vi "Write SA Pin.vi"(8 "error in (no error)":errorcluster, 10 "SA Pin":string, 11 "SpecAn_IM3 in":refnum<class "SpecAn_IM3.lvclass">) -> (0 "error out":errorcluster, 3 "SpecAn_IM3 out":refnum<class "SpecAn_IM3.lvclass">)   [LabVIEW 2018, in "SeqAuto Evaluations.lvlib" / "SpecAn_IM3.lvclass"]
uses:
  SpecAn_IM3.lvclass
  SpecAn_IM3.lvclass/SpecAn_IM3.ctl
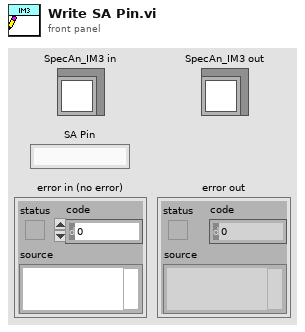
[diagram p1: front panel]
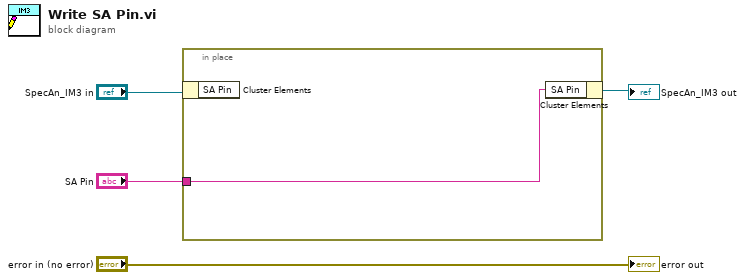
[diagram p0: block diagram]
diagram:
  n1 = in-place {
    in-place-border: "SA Pin" -> [w5]
    n2 = in-place-cluster #1("SpecAn_IM3 in") -> ()  [unwired: 1 out]
    n3 = in-place-cluster #1("SA Pin"=w5) -> (→"SpecAn_IM3 out":refnum<class "SpecAn_IM3.lvclass">)
  }
  "error out" <- "error in (no error)"
